vi "SequenceAcquisition.vi"() -> ()   [LabVIEW 2015]
uses:
  <vilib>/Platform/TimedLoop/XDataNode/timing_clust.ctl
  <vilib>/Platform/TimedLoop/XDataNode/nitl_modes.ctl
  <vilib>/Platform/TimedLoop/XDataNode/wakeup.ctl
  <vilib>/platform/TimedLoop/XDataNode/XDataNode.xnode
  <vilib>/Platform/TimedLoop/XDataNode/XDNodeRunTimeDep.lvlib
panel:
  out "LiveCaptureContinuous":bool
  in  "Stop program":bool
  in  "?":enum32{"IC control", "Data analysis"}(tab)
  in  "ICImagingControl":refnum<k7>(container)
  out "Waveform Chart":i32(graph)
  out "loop index":i32
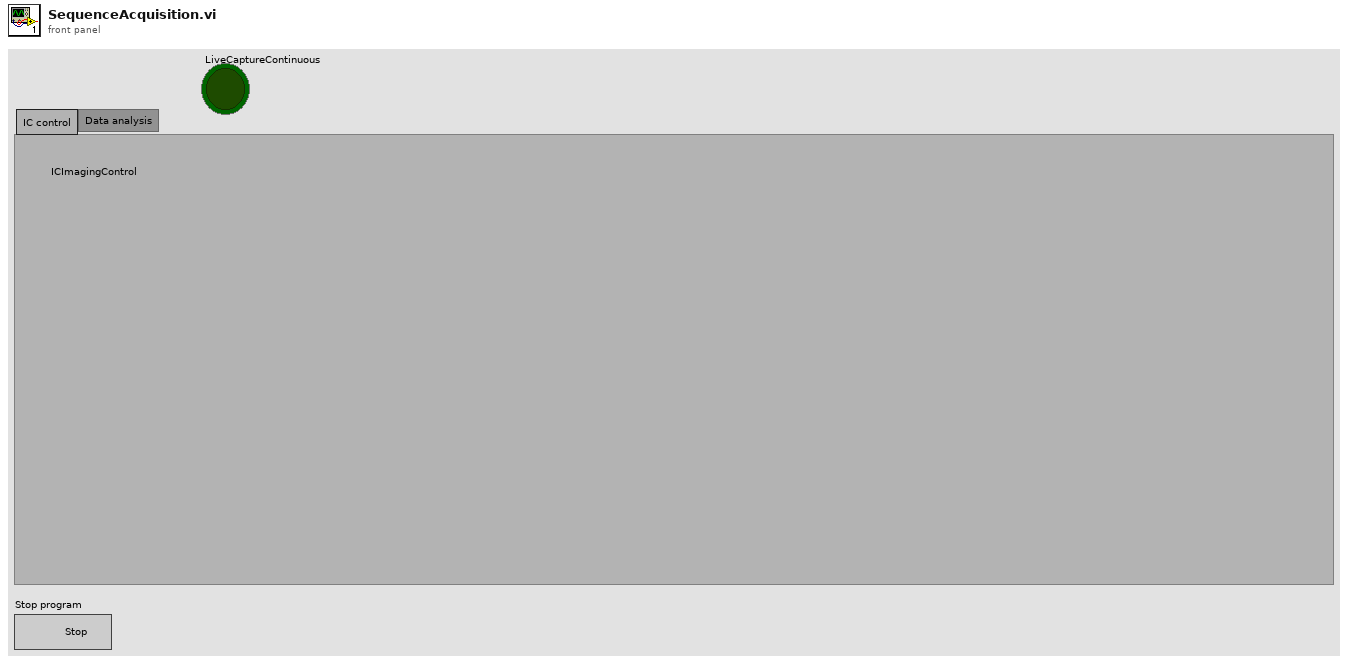
[diagram p1: front panel]
types:
  T1 = typedef "XDNodeRunTimeDep.lvlib/timing_clust.ctl" = cluster{"Expected End [f-1]":u64, "Actual End [f-1]":u64, "Finished Late? [f-1]":bool, "Expected End [i-1]":u64, "Actual End [i-1]":u64, "Finished Late? [i-1]":bool, "Expected Start [i]":u64, "Actual Start [i]":u64, "Expected Start [f]":u64, "Actual Start [f]":u64, "Source Name":string, "Structure Name":string, "Period":i64, "Deadline":i64, "Offset":i64, "Start":i64, "Priority":i32, "Timeout":i32, "Mode":T2, "Wakeup Reason":T3, "Error":errorcluster, "Source Type":string, "Secondary Source Type":string, "Global End Time":u64, "Global Start Time":u64, "Frame Duration":u64, "Iteration Duration":u64, "Assigned CPU":i32, "I/O Scan Engine Mode":u32}
  T2 = typedef "XDNodeRunTimeDep.lvlib/nitl_modes.ctl" = enum32{"No Change", "Process missed periods, maintain original phase", "Discard missed periods, maintain original phase", "Process missed periods, ignore original phase", "Discard missed periods, ignore original phase"}
  T3 = typedef "XDNodeRunTimeDep.lvlib/wakeup.ctl" = enum32{"Normal", "Aborted", "Asynchronous wakeup", "Timing source error", "Timed loop error", "Timeout"}
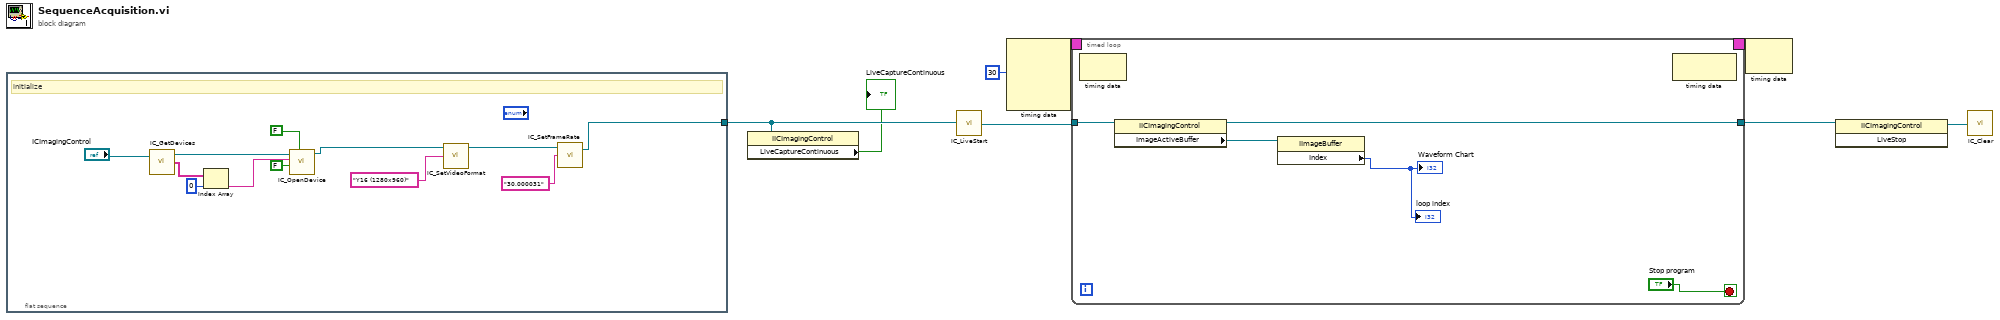
[diagram p0: block diagram]
diagram:
  n1 = flat-sequence {
    tunnel: [w10] -> w5
    frame #0 {
      # "initialize"
      n2 = call <userlib>:"IC_GetDevices.vi"("ICImagingControl In"="ICImagingControl") -> ("ICImagingControl Out"=w17:refnum<k7>, "Devices"=w19:string[])  [unwired: 1 in, 1 out]
      n3 = Index Array(array=w19, index=0) -> (element=w16:string)
      n4 = call <userlib>:"IC_OpenDevice.vi"("Color"=FALSE, "Live"=FALSE, "Device"=w16, "ICImagingControl In"=w17) -> ("ICImagingControl Out"=w13:refnum<k7>)  [unwired: 2 in, 5 out]
      n5 = call <userlib>:"IC_SetVideoFormat.vi"("VideoFormat"="Y16 (1280x960)", "ICImagingControl In"=w13) -> ("ICImagingControl Out"=w11:refnum<k7>)  [unwired: 1 in, 2 out]
      n6 = call <userlib>:"IC_SetFrameRate.vi"("FrameRate"="30,000031", "ICImagingControl In"=w11) -> ("ICImagingControl Out"=w10:refnum<k7>)  [unwired: 1 in, 1 out]
    }
  }
  n7 = property class="IICImagingControl"(reference=w5) -> ("LiveCaptureContinuous"=→"LiveCaptureContinuous":bool)  [unwired: 1 in, 2 out]
  n8 = call <userlib>:"IC_LiveStart.vi"("ICImagingControl 3"=w5) -> ("ICImagingControl 2"=w6:refnum<k7>)
  n9 = node-c288(i64 30 ("Period")) -> (w3:T1)  [unwired: 3 in]
  n10 = timed-loop {
    tunnel: w6 -> [w24]
    tunnel: [w23] -> w7
    timing: w3 -> [_]
    timing-out: [_] -> w2
    stop <- "Stop program" stop-if-true
    n11 = node-c288() -> ()  [unwired: 1 in, 1 out]
    n12 = property class="IICImagingControl"(reference=w24) -> (reference out=w23:refnum<k7>, "ImageActiveBuffer"=w22:refnum<k7>)  [unwired: 1 in, 1 out]
    n13 = property class="IImageBuffer"(reference=w22) -> ("Index"=→"loop index" →"Waveform Chart":i32)  [unwired: 1 in, 2 out]
    n14 = node-c288() -> ()  [unwired: 1 in, 1 out]
  }
  n15 = node-c288(w2) -> ()  [unwired: 1 out]
  n16 = invoke class="IICImagingControl" method="LiveStop"(reference=w7) -> (reference out=w8:refnum<k7>)  [unwired: 2 in, 2 out]
  n17 = call <userlib>:"IC_Clear.vi"("ICImagingControl 2"=w8) -> ()  [unwired: 1 out]
